vi "PicoScope2000IsReady.vi"(8 "error in (no error)":errorcluster, 11 "handle in":i16) -> (0 "error out":errorcluster, 3 "handle out":i16, 6 "ready":i16)   [LabVIEW 2010]
doc: "Calls ps5000aIsReady"
uses:
  ps2000.dll
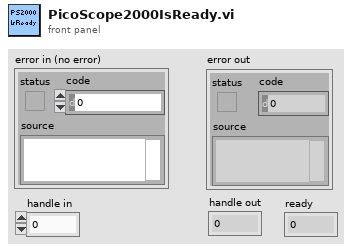
[diagram p1: front panel]
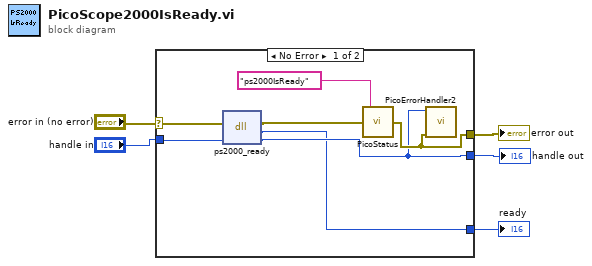
[diagram p0: block diagram]
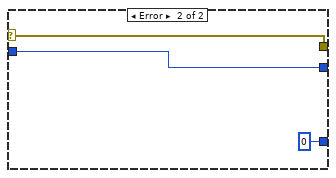
[diagram p2: hidden frame]
diagram:
  n1 = case shown="No Error" "error in (no error)" {
    selector: "error in (no error)" -> [w7 w14]
    tunnel: "handle in" -> [w6 w15]
    tunnel: [w10 w15] -> w5
    tunnel: [w11 w14] -> w4
    tunnel: [w8 i16 0 ("ready")] -> w3
    frame No Error {
      n2 = dll-call lib="PS2000.dll" fn="ps2000_ready"(error in=w7, "handle"=w6) -> (error out=w9:errorcluster, "return type"=w8:i16, "handle"=w10:i16)  [unwired: 2 in, 1 out]
      n3 = call "PicoStatus.vi"("error in"=w9, "source"="ps2000IsReady") -> ("error out"=w11:errorcluster)  [unwired: 1 in]
      n4 = call "PicoErrorHandler2.vi"("error in (no error)"=w11, "handle In"=w10) -> ()  [unwired: 9 in, 1 out]
    }
    frame Error {
    }
  }
  "error out" <- w4
  "handle out" <- w5
  "ready" <- w3
